vi "main-rev.vi"() -> ()   [LabVIEW 2020]
uses:
  GlobalDeviceNum1.vi
  support/Message Queue/Message Queue.lvlib
  support/User Event - Stop/User Event - Stop.lvlib
  setup/support/rev_setup.lvlib
  rev_meas/rev_meas.lvlib
panel:
  in  "EM设置":bool
  in  "HW设置":bool
  in  "退出":bool
  in  "开始":bool
  in  "选项卡控件":enum32{"当前结果", "记录结果", "分析结果"}(tab)
  in  "T1":bool
  in  "T2":bool
  in  "当前混响结果":i32(listbox)
  out "波形图":dbl[](graph)
  in  "deletelineT1":bool
  in  "clearlistT1":bool
  in  "deletelineT2":bool
  in  "clearlistT2":bool
  in  "T1结果":i32(listbox)
  in  "T2结果":i32(listbox)
  in  "All results":i32(listbox)
  in  "analysis":bool
  out "欢迎":string="欢迎使用"
  out "日期/时间字符串":string
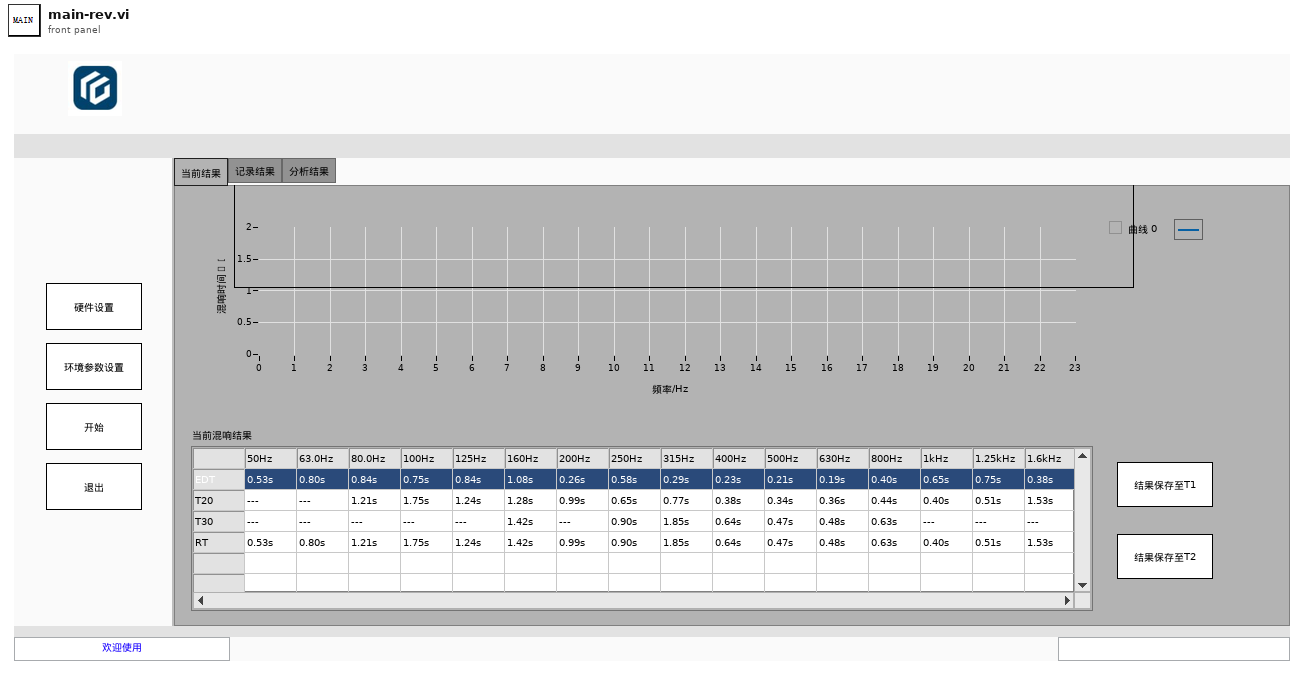
[diagram p1: front panel]
types:
  T1 = typedef "Message Queue.lvlib/All Message Queues.ctl" = cluster{"UI":refnum<queue>, "采集":refnum<queue>, "记录":refnum<queue>}
  T2 = cluster{"T1":dbl[], "T2":dbl[], "A1":dbl[], "A2":dbl[], "AT":dbl[], "Aobj":dbl[], "αs":dbl[]}
  T3 = cluster{"T1":string[], "T2":string[], "A1":string[], "A2":string[], "AT":string[], "Aobj":string[], "αs":string[]}
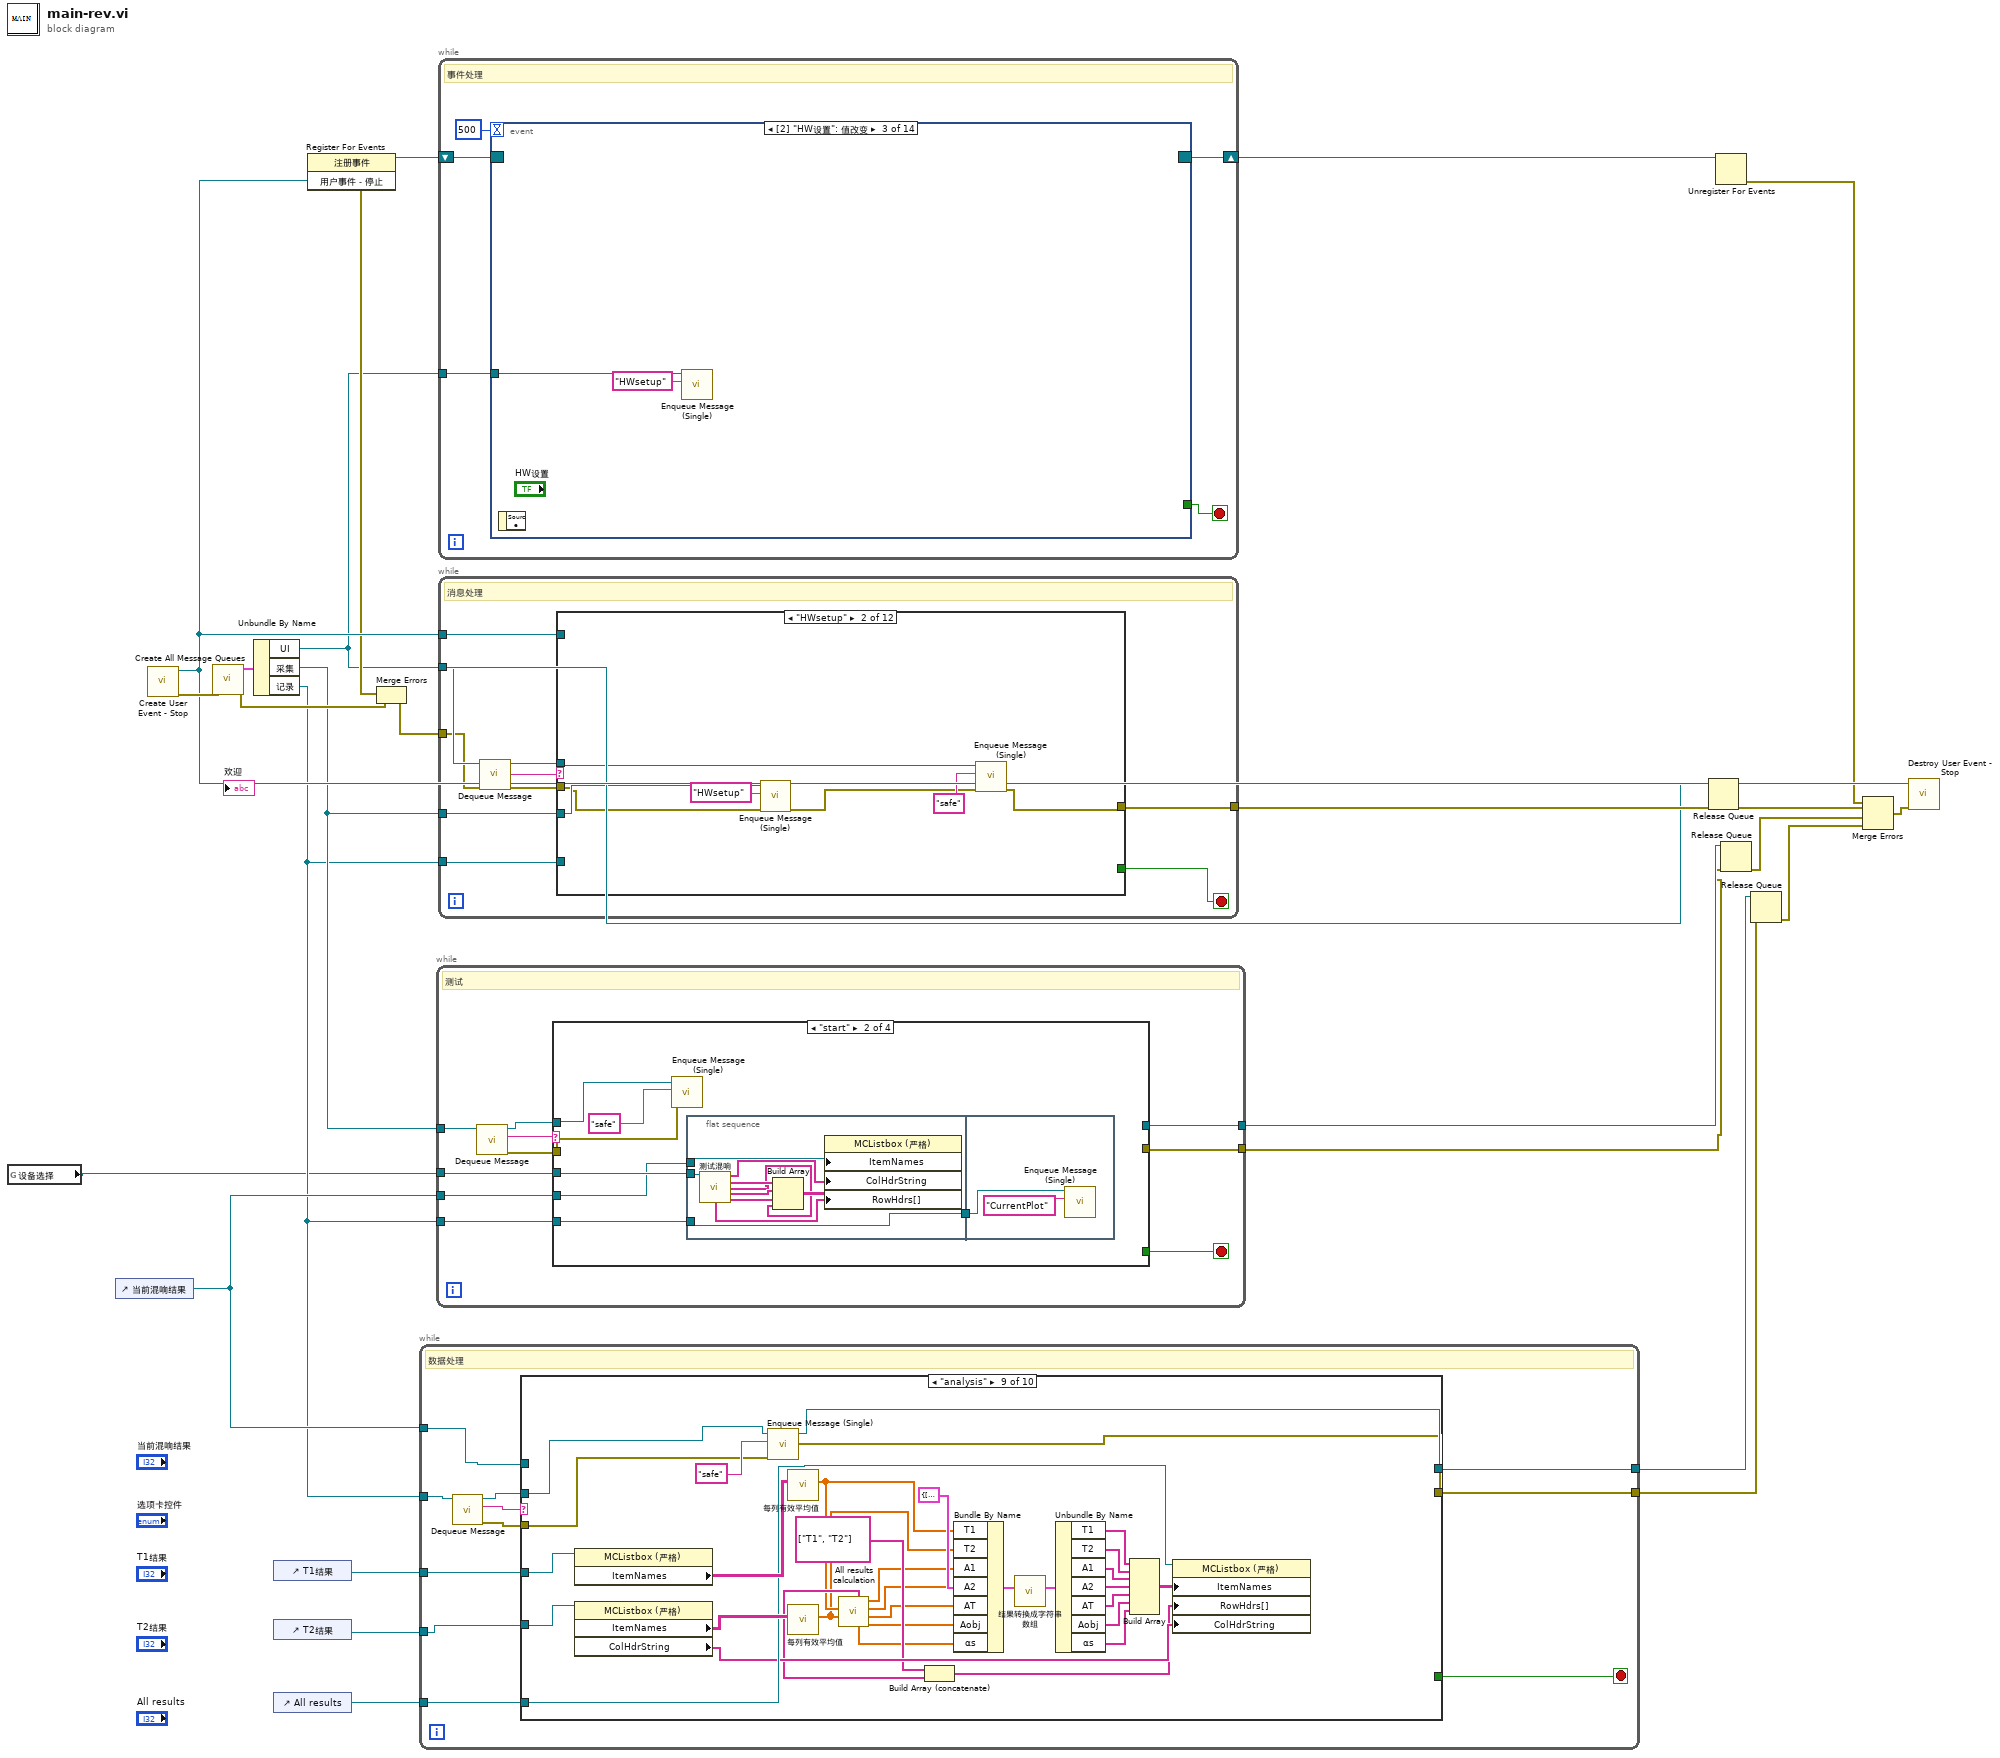
[diagram p0: block diagram]
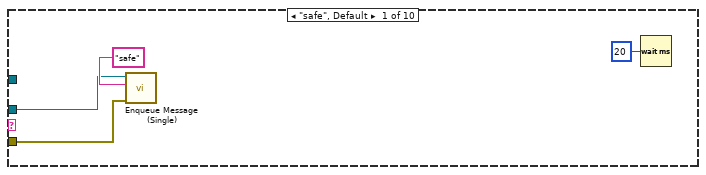
[diagram p2: hidden frame]
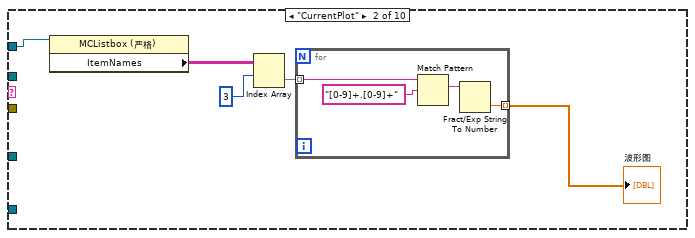
[diagram p3: hidden frame]
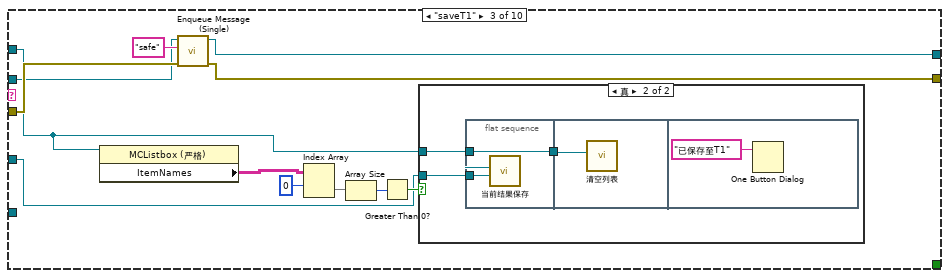
[diagram p4: hidden frame]
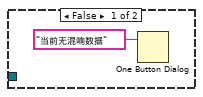
[diagram p5: hidden frame]
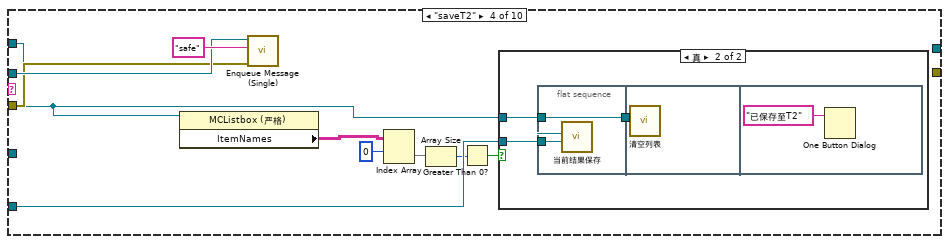
[diagram p6: hidden frame]
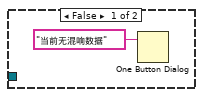
[diagram p7: hidden frame]
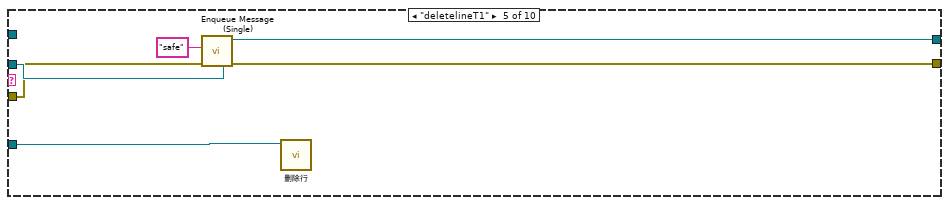
[diagram p8: hidden frame]
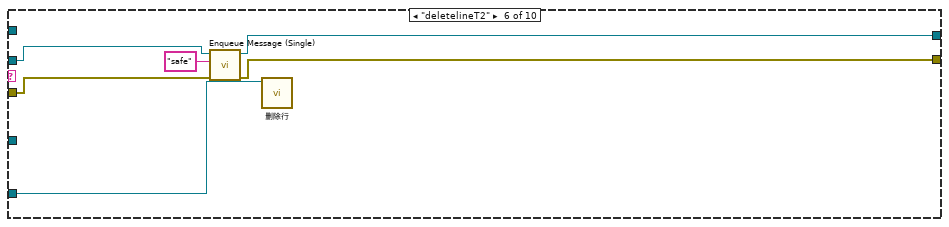
[diagram p9: hidden frame]
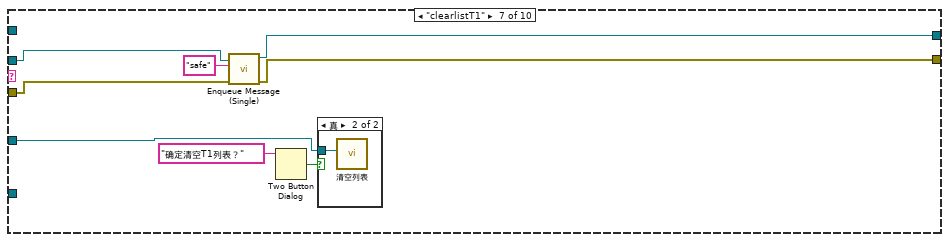
[diagram p10: hidden frame]
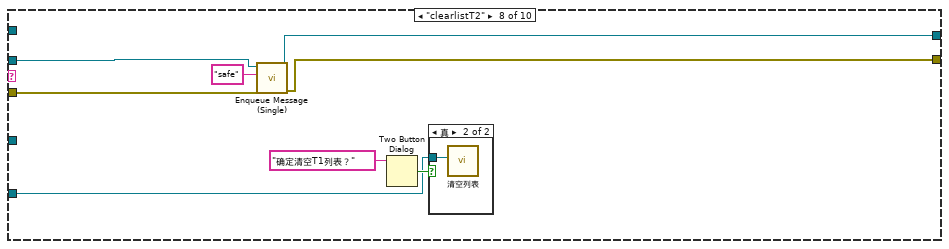
[diagram p12: hidden frame]
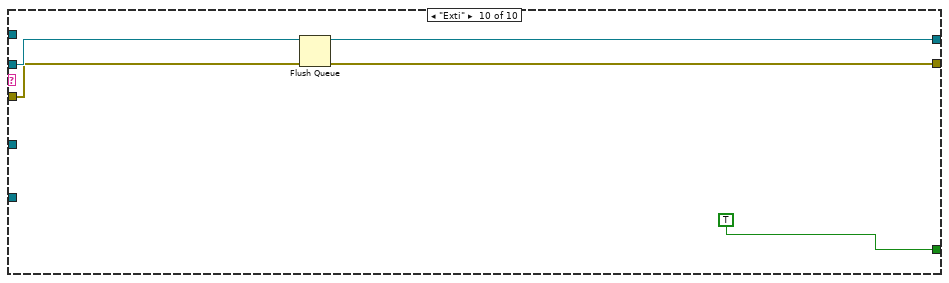
[diagram p14: hidden frame]
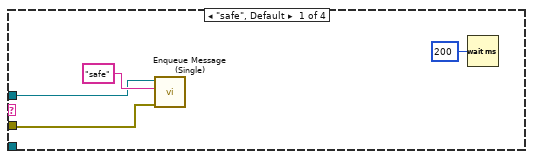
[diagram p15: hidden frame]
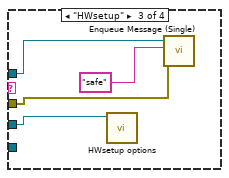
[diagram p16: hidden frame]
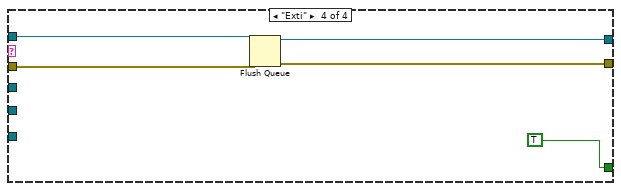
[diagram p17: hidden frame]
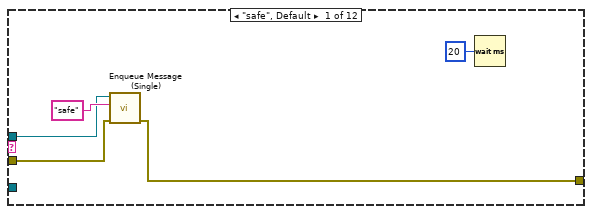
[diagram p18: hidden frame]
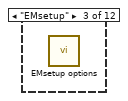
[diagram p19: hidden frame]
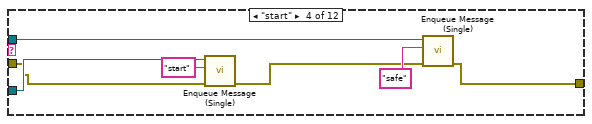
[diagram p20: hidden frame]
diagram:
  n1 = global read "GlobalDeviceNum1.vi" "设备选择"() -> (w1:refnum<visa-resource-name>)
  n2 = control-ref of="当前混响结果"() -> (w6:refnum<vi>)
  n3 = call "Create User Event - Stop.vi"() -> ("error out"=w24:cluster{"状态":bool, "代码":i32, "源":string}, "用户事件－停止"=w23:refnum<user-event>)  [unwired: 10 in]
  n4 = call "Create All Message Queues.vi"("error in (no error)"=w24) -> ("error out"=w21:cluster{"状态":bool, "代码":i32, "源":string}, "消息队列输出"=w26:T1)  [unwired: 9 in]
  n5 = Unbundle By Name(w26) -> ("UI"=w17:refnum<queue>, "采集"=w16:refnum<queue>, "记录"=w3:refnum<queue>)
  n6 = control-ref of="T1结果"() -> (w5:refnum<vi>)
  n7 = control-ref of="T2结果"() -> (w4:refnum<vi>)
  n8 = control-ref of="All results"() -> (w2:refnum<vi>)
  n9 = register-events(w23) -> (reference out=w25:refnum<event-registration>, error out=w20:errorcluster)  [unwired: 2 in]
  n10 = Merge Errors(w20, w21) -> (w19:errorcluster)
  n11 = while {
    tunnel: w3 -> [w36]
    tunnel: w6 -> [w34]
    tunnel: [w31] -> w10
    tunnel: [w30] -> w7
    tunnel: w5 -> [w29]
    tunnel: w4 -> [w28]
    tunnel: w2 -> [w27]
    stop <- w35 stop-if-true
    # "数据处理"
    n12 = call "Dequeue Message.vi"("消息队列"=w36) -> ("error out"=w32:cluster{"状态":bool, "代码":i32, "源":string}, "消息"=w37:string, "消息队列副本"=w33:refnum<queue>)  [unwired: 7 in, 1 out]
    n13 = case shown="\"analysis\"" w37 {
      tunnel: [_ _ _ _ _ _ _ _ _ TRUE] -> w35
      tunnel: w34 -> [_ w46 w51 w76 _ _ _ _ _ _]
      tunnel: w33 -> [w39 _ w58 w79 w93 w99 w105 w113 w149 w154]
      tunnel: w32 -> [w38 _ w61 w78 w92 w98 w104 w114 w148 w152]
      tunnel: [_ _ w60 _ w91 w97 w107 w116 w147 w153] -> w31
      tunnel: [_ _ w59 _ w90 w96 w106 w115 w146 w151] -> w30
      tunnel: w29 -> [_ _ w52 _ w89 _ w101 _ w145 _]
      tunnel: w28 -> [_ _ _ w77 _ w95 _ w110 w144 _]
      tunnel: w27 -> [_ _ _ _ _ _ _ _ w141 _]
      frame "safe", Default {
        n14 = call "Enqueue Message (Single).vi"("error in (no error)"=w38, "消息"="safe", "消息队列"=w39) -> ()  [unwired: 7 in, 2 out]
        n15 = Wait (ms)(milliseconds to wait=u32 20 ("等待时间（毫秒）")) -> ()  [unwired: 1 out]
      }
      frame "CurrentPlot" {
        n16 = property class="MCListbox (严格)"(reference=w46) -> ("ItemNames"=w45:string[][])  [unwired: 1 in, 2 out]
        n17 = Index Array(array=w45, index (row)=3 ("索引 (行)")) -> (element=w43:string[])  [unwired: 1 in]
        n18 = for {
          tunnel: w43 -> [w50] mode=indexing
          tunnel: [w47] -> w42 mode=indexing
          n19 = Match Pattern(string=w50, regular expression="[0-9]+.[0-9]+" ("正则表达式")) -> (match substring=w48:string)  [unwired: 1 in, 3 out]
          n20 = Fract/Exp String To Number(string=w48) -> (number=w47:dbl)  [unwired: 3 in, 1 out]
        }
        "波形图" <- w42
      }
      frame "saveT1" {
        n21 = property class="MCListbox (严格)"(reference=w51) -> ("ItemNames"=w56:string[][])  [unwired: 1 in, 2 out]
        n22 = call "Enqueue Message (Single).vi"("error in (no error)"=w61, "消息"="safe", "消息队列"=w58) -> ("error out"=w59:cluster{"状态":bool, "代码":i32, "源":string}, "消息队列副本"=w60:refnum<queue>)  [unwired: 7 in]
        n23 = Index Array(array=w56, index (row)=0 ("索引 (行)")) -> (element=w54:string[])  [unwired: 1 in]
        n24 = Array Size(array=w54) -> (size(s)=w57:i32)
        n25 = Greater Than 0?(x=w57) -> (x > 0?=w53:bool)
        n26 = case shown="真" w53 {
          tunnel: w52 -> [_ w66]
          tunnel: w51 -> [_ w65]
          frame False {
            n27 = One Button Dialog(message="当前无混响数据" ("消息")) -> ()  [unwired: 1 in, 1 out]
          }
          frame True {
            n28 = flat-sequence {
              tunnel: w66 -> [w68]
              tunnel: w65 -> [w67]
              tunnel: [w67] -> w64
              tunnel: w64 -> [w69]
              frame #0 {
                n29 = call "当前结果保存.vi"("列表2"=w68, "列表1"=w67) -> ()  [unwired: 10 in]
              }
              frame #1 {
                n30 = call "清空列表.vi"("列表"=w69) -> ()  [unwired: 11 in]
              }
              frame #2 {
                n31 = One Button Dialog(message="已保存至T1" ("消息")) -> ()  [unwired: 1 in, 1 out]
              }
            }
          }
        }
      }
      frame "saveT2" {
        n32 = property class="MCListbox (严格)"(reference=w76) -> ("ItemNames"=w74:string[][])  [unwired: 1 in, 2 out]
        n33 = call "Enqueue Message (Single).vi"("error in (no error)"=w78, "消息"="safe", "消息队列"=w79) -> ()  [unwired: 7 in, 2 out]
        n34 = Index Array(array=w74, index (row)=0 ("索引 (行)")) -> (element=w72:string[])  [unwired: 1 in]
        n35 = Array Size(array=w72) -> (size(s)=w75:i32)
        n36 = Greater Than 0?(x=w75) -> (x > 0?=w71:bool)
        n37 = case shown="真" w71 {
          tunnel: w77 -> [_ w84]
          tunnel: w76 -> [_ w83]
          frame False {
            n38 = One Button Dialog(message="当前无混响数据" ("消息")) -> ()  [unwired: 1 in, 1 out]
          }
          frame True {
            n39 = flat-sequence {
              tunnel: w84 -> [w86]
              tunnel: w83 -> [w85]
              tunnel: [w85] -> w82
              tunnel: w82 -> [w87]
              frame #0 {
                n40 = call "当前结果保存.vi"("列表2"=w86, "列表1"=w85) -> ()  [unwired: 10 in]
              }
              frame #1 {
                n41 = call "清空列表.vi"("列表"=w87) -> ()  [unwired: 11 in]
              }
              frame #2 {
                n42 = One Button Dialog(message="已保存至T2" ("消息")) -> ()  [unwired: 1 in, 1 out]
              }
            }
          }
        }
      }
      frame "deletelineT1" {
        n43 = call "Enqueue Message (Single).vi"("error in (no error)"=w92, "消息"="safe", "消息队列"=w93) -> ("error out"=w90:cluster{"状态":bool, "代码":i32, "源":string}, "消息队列副本"=w91:refnum<queue>)  [unwired: 7 in]
        n44 = call "删除行.vi"("列表"=w89) -> ()  [unwired: 11 in]
      }
      frame "deletelineT2" {
        n45 = call "Enqueue Message (Single).vi"("error in (no error)"=w98, "消息"="safe", "消息队列"=w99) -> ("error out"=w96:cluster{"状态":bool, "代码":i32, "源":string}, "消息队列副本"=w97:refnum<queue>)  [unwired: 7 in]
        n46 = call "删除行.vi"("列表"=w95) -> ()  [unwired: 11 in]
      }
      frame "clearlistT1" {
        n47 = call "Enqueue Message (Single).vi"("error in (no error)"=w104, "消息"="safe", "消息队列"=w105) -> ("error out"=w106:cluster{"状态":bool, "代码":i32, "源":string}, "消息队列副本"=w107:refnum<queue>)  [unwired: 7 in]
        n48 = Two Button Dialog(message="确定清空T1列表？" ("消息")) -> (T button?=w102:bool)  [unwired: 2 in]
        n49 = case shown="真" w102 {
          tunnel: w101 -> [_ w109]
          frame False {
          }
          frame True {
            n50 = call "清空列表.vi"("列表"=w109) -> ()  [unwired: 11 in]
          }
        }
      }
      frame "clearlistT2" {
        n51 = call "Enqueue Message (Single).vi"("error in (no error)"=w114, "消息"="safe", "消息队列"=w113) -> ("error out"=w115:cluster{"状态":bool, "代码":i32, "源":string}, "消息队列副本"=w116:refnum<queue>)  [unwired: 7 in]
        n52 = Two Button Dialog(message="确定清空T1列表？" ("消息")) -> (T button?=w111:bool)  [unwired: 2 in]
        n53 = case shown="真" w111 {
          tunnel: w110 -> [_ w118]
          frame False {
          }
          frame True {
            n54 = call "清空列表.vi"("列表"=w118) -> ()  [unwired: 11 in]
          }
        }
      }
      frame "analysis" {
        n55 = property class="MCListbox (严格)"(reference=w145) -> ("ItemNames"=w143:string[][])  [unwired: 1 in, 2 out]
        n56 = property class="MCListbox (严格)"(reference=w144) -> ("ItemNames"=w142:string[][], "ColHdrString"=w140:string[])  [unwired: 1 in, 2 out]
        n57 = call "Enqueue Message (Single).vi"("error in (no error)"=w148, "消息"="safe", "消息队列"=w149) -> ("error out"=w146:cluster{"状态":bool, "代码":i32, "源":string}, "消息队列副本"=w147:refnum<queue>)  [unwired: 7 in]
        n58 = call "每列有效平均值.vi"("测试数组"=w143) -> ("平均混响时间"=w136:dbl[])  [unwired: 10 in]
        n59 = call "每列有效平均值.vi"("测试数组"=w142) -> ("平均混响时间"=w135:dbl[])  [unwired: 10 in]
        n60 = call "All results calculation.vi"("平均混响时间T2"=w135, "平均混响时间T1"=w136) -> ("分立吸声体吸声量Aobj"=w131:dbl[], "试件吸声量AT"=w132:dbl[], "混响室吸声量A2"=w133:dbl[], "混响室吸声量A1"=w134:dbl[], "吸声系数αs"=w130:dbl[], "rowhead"=w138:string[])  [unwired: 4 in]
        n61 = Build Array (concatenate)(string[] ["T1", "T2"], w138) -> (w119:string[])
        n62 = Bundle By Name(cluster=T2 {"T1"=[], "T2"=[], "A1"=[], "A2"=[], "AT"=[], "Aobj"=[], "αs"=[]} ("结果数据数组簇"), "T1"=w136, "T2"=w135, "A1"=w134, "A2"=w133, "AT"=w132, "Aobj"=w131, "αs"=w130) -> (w129:T2)
        n63 = call "结果转换成字符串数组.vi"("结果数据数组簇"=w129) -> ("结果字符串数组簇"=w128:T3)  [unwired: 10 in]
        n64 = Unbundle By Name(w128) -> ("T1"=w127:string[], "T2"=w126:string[], "A1"=w125:string[], "A2"=w124:string[], "AT"=w123:string[], "Aobj"=w122:string[], "αs"=w121:string[])
        n65 = Build Array(w127, w126, w125, w124, w123, w122, w121) -> (w120:string[][])
        n66 = property class="MCListbox (严格)"(reference=w141, "ItemNames"=w120, "RowHdrs[]"=w119, "ColHdrString"=w140) -> ()  [unwired: 1 in, 2 out]
      }
      frame "Exti" {
        n67 = Flush Queue(queue=w154, error in (no error)=w152) -> (queue out=w153:refnum<queue>, error out=w151:errorcluster)  [unwired: 1 out]
      }
    }
  }
  n68 = while {
    tunnel: w16 -> [w165]
    tunnel: w1 -> [w162]
    tunnel: w6 -> [w159]
    tunnel: [w158] -> w12
    tunnel: [w157] -> w8
    tunnel: w3 -> [w156]
    stop <- w160 stop-if-true
    # "测试"
    n69 = call "Dequeue Message.vi"("消息队列"=w165) -> ("error out"=w163:cluster{"状态":bool, "代码":i32, "源":string}, "消息"=w161:string, "消息队列副本"=w164:refnum<queue>)  [unwired: 7 in, 1 out]
    n70 = case shown="\"start\"" w161 {
      tunnel: w164 -> [w167 w176 w190 w196]
      tunnel: w163 -> [w166 w175 w189 w194]
      tunnel: w162 -> [_ w173 w192 _]
      tunnel: [_ _ _ TRUE] -> w160
      tunnel: w159 -> [_ w172 _ _]
      tunnel: [_ _ _ w195] -> w158
      tunnel: [_ _ _ w193] -> w157
      tunnel: w156 -> [_ w170 _ _]
      frame "safe", Default {
        n71 = call "Enqueue Message (Single).vi"("error in (no error)"=w166, "消息"="safe", "消息队列"=w167) -> ()  [unwired: 7 in, 2 out]
        n72 = Wait (ms)(milliseconds to wait=u32 200 ("等待时间（毫秒）")) -> ()  [unwired: 1 out]
      }
      frame "start" {
        n73 = call "Enqueue Message (Single).vi"("error in (no error)"=w175, "消息"="safe", "消息队列"=w176) -> ()  [unwired: 7 in, 2 out]
        n74 = flat-sequence {
          tunnel: w173 -> [w184]
          tunnel: w172 -> [w185]
          tunnel: [w179] -> w171
          tunnel: w170 -> [w179]
          tunnel: w171 -> [w188]
          frame #0 {
            n75 = call "测试混响.vi"("VISA资源名称"=w184) -> ("频率输出"=w178:string[], "EDT输出"=w183:string[], "RT result"=w180:string[], "T20输出"=w182:string[], "rowhead"=w177:string[], "T30输出"=w181:string[])  [unwired: 9 in]
            n76 = Build Array(w183, w182, w181, w180) -> (w186:string[][])
            n77 = property class="MCListbox (严格)"(reference=w185, "ItemNames"=w186, "ColHdrString"=w178, "RowHdrs[]"=w177) -> ()  [unwired: 1 in, 2 out]
          }
          frame #1 {
            n78 = call "Enqueue Message (Single).vi"("消息"="CurrentPlot", "消息队列"=w188) -> ()  [unwired: 8 in, 2 out]
          }
        }
      }
      frame "HWsetup" {
        n79 = call "HWsetup options.vi"("设备选择"=w192) -> ()  [unwired: 11 in]
        n80 = call "Enqueue Message (Single).vi"("error in (no error)"=w189, "消息"="safe", "消息队列"=w190) -> ()  [unwired: 7 in, 2 out]
      }
      frame "Exti" {
        n81 = Flush Queue(queue=w196, error in (no error)=w194) -> (queue out=w195:refnum<queue>, error out=w193:errorcluster)  [unwired: 1 out]
      }
    }
  }
  n82 = while {
    tunnel: w17 -> [w201]
    shift-right: [w199] -> w22
    shift-left: w25 -> [w200]
    stop <- w202 stop-if-true
    # "事件处理"
    n83 = event shown="[2] \"HW设置\": 值改变" {
      selector: w200 -> [_ _ _ _ _ _ _ _ _ _ _ _ _ _]
      dyn-events: [_ _ _ _ _ _ _ _ _ _ _ _ _ _] -> w199
      timeout: 500 -> [_ _ _ _ _ _ _ _ _ _ _ _ _ _]
      tunnel: [_ w207 _ _ _ _ TRUE _ _ _ _ _ _ _] -> w202
      tunnel: w201 -> [_ w204 w209 w210 w213 w215 _ w218 w220 w222 w224 w226 w228 w230]
      event Timeout {
        n84 = event-data() -> ()  [unwired: 1 in, 3 out]
        n85 = Format Date/Time String() -> (date/time string=→"日期/时间字符串":string)  [unwired: 3 in]
      }
      event Panel Close? {
        w207 = TRUE ("放弃？")
        n86 = event-data() -> ()  [unwired: 1 in, 4 out]
        n87 = call "Enqueue Message (Single).vi"("优先消息？ (F)"=TRUE, "消息"="Exti", "消息队列"=w204) -> ()  [unwired: 7 in, 2 out]
        n88 = event-data("Discard?"=w207) -> ()  [unwired: 1 in, 1 out]
      }
      event "HW设置": Value Change {
        n89 = event-data() -> ()  [unwired: 1 in, 1 out]
        n90 = call "Enqueue Message (Single).vi"("消息"="HWsetup", "消息队列"=w209) -> ()  [unwired: 8 in, 2 out]
      }
      event "EM设置": Value Change {
        n91 = event-data() -> ()  [unwired: 1 in, 1 out]
        n92 = call "Enqueue Message (Single).vi"("消息"="EMsetup", "消息队列"=w210) -> ()  [unwired: 8 in, 2 out]
      }
      event "开始": Value Change {
        n93 = event-data() -> ()  [unwired: 1 in, 1 out]
        n94 = call "Enqueue Message (Single).vi"("消息"="start", "消息队列"=w213) -> ()  [unwired: 8 in, 2 out]
      }
      event "退出": Value Change {
        n95 = event-data() -> ()  [unwired: 1 in, 1 out]
        n96 = call "Enqueue Message (Single).vi"("优先消息？ (F)"=TRUE, "消息"="Exti", "消息队列"=w215) -> ()  [unwired: 7 in, 2 out]
      }
      event User Event {
        n97 = event-data() -> ()  [unwired: 1 in, 1 out]
      }
      event "T1": Value Change {
        n98 = event-data() -> ()  [unwired: 1 in, 1 out]
        n99 = call "Enqueue Message (Single).vi"("消息"="saveT1", "消息队列"=w218) -> ()  [unwired: 8 in, 2 out]
      }
      event "T2": Value Change {
        n100 = event-data() -> ()  [unwired: 1 in, 1 out]
        n101 = call "Enqueue Message (Single).vi"("消息"="saveT2", "消息队列"=w220) -> ()  [unwired: 8 in, 2 out]
      }
      event "deletelineT1": Value Change {
        n102 = event-data() -> ()  [unwired: 1 in, 1 out]
        n103 = call "Enqueue Message (Single).vi"("消息"="deletelineT1", "消息队列"=w222) -> ()  [unwired: 8 in, 2 out]
      }
      event "deletelineT2": Value Change {
        n104 = event-data() -> ()  [unwired: 1 in, 1 out]
        n105 = call "Enqueue Message (Single).vi"("消息"="deletelineT2", "消息队列"=w224) -> ()  [unwired: 8 in, 2 out]
      }
      event "clearlistT1": Value Change {
        n106 = event-data() -> ()  [unwired: 1 in, 1 out]
        n107 = call "Enqueue Message (Single).vi"("消息"="clearlistT1", "消息队列"=w226) -> ()  [unwired: 8 in, 2 out]
      }
      event "clearlistT2": Value Change {
        n108 = event-data() -> ()  [unwired: 1 in, 1 out]
        n109 = call "Enqueue Message (Single).vi"("消息"="clearlistT2", "消息队列"=w228) -> ()  [unwired: 8 in, 2 out]
      }
      event "analysis": Value Change {
        n110 = event-data() -> ()  [unwired: 1 in, 1 out]
        n111 = call "Enqueue Message (Single).vi"("消息"="analysis", "消息队列"=w230) -> ()  [unwired: 8 in, 2 out]
      }
    }
  }
  n112 = while {
    tunnel: w17 -> [w241]
    tunnel: w23 -> [w239]
    tunnel: w19 -> [w237]
    tunnel: [w236] -> w18
    tunnel: w16 -> [w233]
    tunnel: w3 -> [w232]
    stop <- w238 stop-if-true
    # "消息处理"
    n113 = call "Dequeue Message.vi"("error in (no error)"=w237, "消息队列"=w241) -> ("error out"=w234:cluster{"状态":bool, "代码":i32, "源":string}, "消息"=w240:string, "消息队列副本"=w235:refnum<queue>)  [unwired: 6 in, 1 out]
    n114 = case shown="\"HWsetup\"" w240 {
      tunnel: w239 -> [_ _ _ _ _ _ _ _ _ _ _ w316]
      tunnel: [_ _ _ _ _ _ _ _ _ _ _ TRUE] -> w238
      tunnel: [w243 w247 _ w258 w261 _ w274 _ w287 w297 w301 w314] -> w236
      tunnel: w235 -> [w245 w250 _ w259 w264 w270 w277 w283 w289 w295 w302 w308]
      tunnel: w234 -> [w244 w248 _ w256 w262 w268 w275 w282 w288 w296 w303 _]
      tunnel: w233 -> [_ w249 _ w257 _ _ _ _ _ _ _ w313]
      tunnel: w232 -> [_ _ _ _ w263 w269 w276 w281 w290 w294 w304 w311]
      frame "safe", Default {
        n115 = call "Enqueue Message (Single).vi"("error in (no error)"=w244, "消息"="safe", "消息队列"=w245) -> ("error out"=w243:cluster{"状态":bool, "代码":i32, "源":string})  [unwired: 7 in, 1 out]
        n116 = Wait (ms)(milliseconds to wait=u32 20 ("等待时间（毫秒）")) -> ()  [unwired: 1 out]
      }
      frame "HWsetup" {
        n117 = call "Enqueue Message (Single).vi"("error in (no error)"=w248, "消息"="HWsetup", "消息队列"=w249) -> ("error out"=w252:cluster{"状态":bool, "代码":i32, "源":string})  [unwired: 7 in, 1 out]
        n118 = call "Enqueue Message (Single).vi"("error in (no error)"=w252, "消息"="safe", "消息队列"=w250) -> ("error out"=w247:cluster{"状态":bool, "代码":i32, "源":string})  [unwired: 7 in, 1 out]
      }
      frame "EMsetup" {
        n119 = call "EMsetup options.vi"() -> ()  [unwired: 12 in]
      }
      frame "start" {
        n120 = call "Enqueue Message (Single).vi"("error in (no error)"=w256, "消息"="start", "消息队列"=w257) -> ("error out"=w255:cluster{"状态":bool, "代码":i32, "源":string})  [unwired: 7 in, 1 out]
        n121 = call "Enqueue Message (Single).vi"("error in (no error)"=w255, "消息"="safe", "消息队列"=w259) -> ("error out"=w258:cluster{"状态":bool, "代码":i32, "源":string})  [unwired: 7 in, 1 out]
      }
      frame "saveT1" {
        n122 = call "Enqueue Message (Single).vi"("error in (no error)"=w262, "消息"="saveT1", "消息队列"=w263) -> ("error out"=w266:cluster{"状态":bool, "代码":i32, "源":string})  [unwired: 7 in, 1 out]
        n123 = call "Enqueue Message (Single).vi"("error in (no error)"=w266, "消息"="safe", "消息队列"=w264) -> ("error out"=w261:cluster{"状态":bool, "代码":i32, "源":string})  [unwired: 7 in, 1 out]
      }
      frame "saveT2" {
        n124 = call "Enqueue Message (Single).vi"("error in (no error)"=w268, "消息"="saveT2", "消息队列"=w269) -> ("error out"=w273:cluster{"状态":bool, "代码":i32, "源":string})  [unwired: 7 in, 1 out]
        n125 = call "Enqueue Message (Single).vi"("error in (no error)"=w273, "消息"="safe", "消息队列"=w270) -> ()  [unwired: 7 in, 2 out]
      }
      frame "deletelineT1" {
        n126 = call "Enqueue Message (Single).vi"("error in (no error)"=w275, "消息"="deletelineT1", "消息队列"=w276) -> ("error out"=w280:cluster{"状态":bool, "代码":i32, "源":string})  [unwired: 7 in, 1 out]
        n127 = call "Enqueue Message (Single).vi"("error in (no error)"=w280, "消息"="safe", "消息队列"=w277) -> ("error out"=w274:cluster{"状态":bool, "代码":i32, "源":string})  [unwired: 7 in, 1 out]
      }
      frame "deletelineT2" {
        n128 = call "Enqueue Message (Single).vi"("error in (no error)"=w282, "消息"="deletelineT2", "消息队列"=w281) -> ("error out"=w286:cluster{"状态":bool, "代码":i32, "源":string})  [unwired: 7 in, 1 out]
        n129 = call "Enqueue Message (Single).vi"("error in (no error)"=w286, "消息"="safe", "消息队列"=w283) -> ()  [unwired: 7 in, 2 out]
      }
      frame "clearlistT1" {
        n130 = call "Enqueue Message (Single).vi"("error in (no error)"=w288, "消息"="clearlistT1", "消息队列"=w290) -> ("error out"=w293:cluster{"状态":bool, "代码":i32, "源":string})  [unwired: 7 in, 1 out]
        n131 = call "Enqueue Message (Single).vi"("error in (no error)"=w293, "消息"="safe", "消息队列"=w289) -> ("error out"=w287:cluster{"状态":bool, "代码":i32, "源":string})  [unwired: 7 in, 1 out]
      }
      frame "clearlistT2" {
        n132 = call "Enqueue Message (Single).vi"("error in (no error)"=w296, "消息"="clearlistT2", "消息队列"=w294) -> ("error out"=w300:cluster{"状态":bool, "代码":i32, "源":string})  [unwired: 7 in, 1 out]
        n133 = call "Enqueue Message (Single).vi"("error in (no error)"=w300, "消息"="safe", "消息队列"=w295) -> ("error out"=w297:cluster{"状态":bool, "代码":i32, "源":string})  [unwired: 7 in, 1 out]
      }
      frame "analysis" {
        n134 = call "Enqueue Message (Single).vi"("error in (no error)"=w303, "消息"="analysis", "消息队列"=w304) -> ("error out"=w307:cluster{"状态":bool, "代码":i32, "源":string})  [unwired: 7 in, 1 out]
        n135 = call "Enqueue Message (Single).vi"("error in (no error)"=w307, "消息"="safe", "消息队列"=w302) -> ("error out"=w301:cluster{"状态":bool, "代码":i32, "源":string})  [unwired: 7 in, 1 out]
      }
      frame "Exti" {
        w309 = "Exti" ("消息")
        n136 = call "Enqueue Message (Single).vi"("优先消息？ (F)"=TRUE, "消息"=w309, "消息队列"=w313) -> ()  [unwired: 7 in, 2 out]
        n137 = call "Enqueue Message (Single).vi"("优先消息？ (F)"=TRUE, "消息"=w309, "消息队列"=w311) -> ()  [unwired: 7 in, 2 out]
        n138 = call "Fire User Event - Stop.vi"("用户事件－停止"=w316) -> ("error out"=w314:cluster{"状态":bool, "代码":i32, "源":string})  [unwired: 10 in]
        n139 = Flush Queue(queue=w308) -> ()  [unwired: 1 in, 3 out]
      }
    }
  }
  n140 = Release Queue(queue=w17, error in (no error)=w18) -> (error out=w13:errorcluster)  [unwired: 1 in, 2 out]
  n141 = Unregister For Events(event registration refnum=w22) -> (error out=w14:errorcluster)  [unwired: 1 in]
  n142 = Release Queue(queue=w12, error in (no error)=w8) -> (error out=w11:errorcluster)  [unwired: 1 in, 2 out]
  n143 = Release Queue(queue=w10, error in (no error)=w7) -> (error out=w9:errorcluster)  [unwired: 1 in, 2 out]
  n144 = Merge Errors(w14, w13, w11, w9) -> (w15:errorcluster)
  n145 = call "Destroy User Event - Stop.vi"("error in (no error)"=w15, "用户事件－停止"=w23) -> ()  [unwired: 9 in, 1 out]
